vi "HSMS Request.vi"(8 "error in (no error)":errorcluster, 10 "SECS-II Class In":refnum<class "SECS-II Class.lvclass">, 11 "HSMS Class in":refnum<class "HSMS Class.lvclass">) -> (0 "error out":errorcluster, 3 "HSMS Class out":refnum<class "HSMS Class.lvclass">)   [LabVIEW 2020, in "SECS Communication.lvlib" / "HSMS Class.lvclass"]
uses:
  HSMS Class.lvclass
  SECS-II Class/SECS-II Class.lvclass
  Command Data.ctl
  HSMS Class.lvclass/HSMS Class.ctl
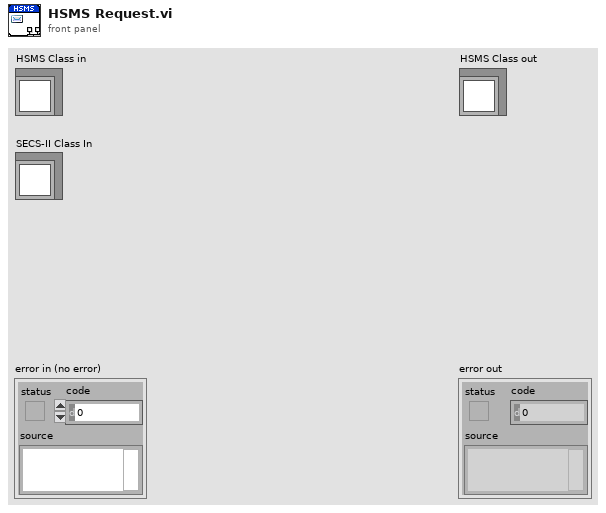
[diagram p1: front panel]
types:
  T1 = typedef "SECS Communication.lvlib/HSMS Class.lvclass/Command Data.ctl" = cluster{"SECS-II Class":refnum<class "SECS-II Class.lvclass">, "Reply Notifier":refnum<notifier>}
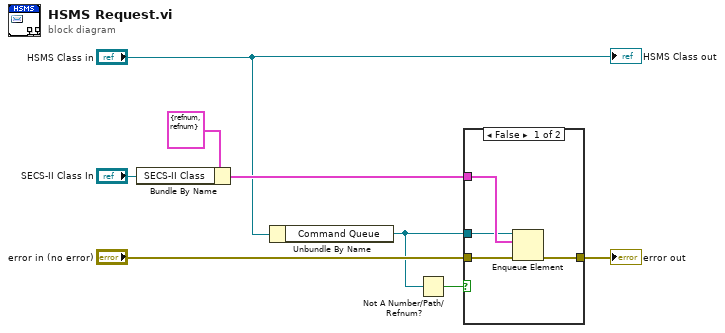
[diagram p0: block diagram]
diagram:
  n1 = Bundle By Name(cluster=T1 {"SECS-II Class"=refnum, "Reply Notifier"=refnum} ("element"), "SECS-II Class"="SECS-II Class In") -> (w6:T1)
  n2 = Unbundle By Name("HSMS Class in") -> ("Command Queue"=w2:refnum<queue>)
  n3 = Not A Number/Path/Refnum?(number/path/refnum=w2) -> (NaN/Path/Refnum?=w1:bool)
  n4 = case shown="False" w1 {
    tunnel: w6 -> [w12 _]
    tunnel: "error in (no error)" -> [w11 w13]
    tunnel: [w10 w13] -> w3
    tunnel: w2 -> [w9 _]
    frame False {
      n5 = Enqueue Element(queue=w9, element=w12, error in (no error)=w11) -> (error out=w10:errorcluster)  [unwired: 1 in, 2 out]
    }
    frame True {
    }
  }
  "error out" <- w3
  "HSMS Class out" <- "HSMS Class in"
